vi "Check for Rx Label Updates.vi"(8 "error in":errorcluster, 9 "labels settings for RT":T1[](array[typedef]) {"Label Timestamp Channel Data Reference" format="%.0x"; "Word Initial Raw Value" format="%032.0f"; "Label Disable/Trigger Channel Reference" format="%.0x"; "parameter driver data"."Tx parameter refs" format="%.0x"; "SDI" format="%02b"; "label" format="%.0o"}, 10 "channel number in":u8, 11 "board handle in":u8) -> (0 "error out":errorcluster, 1 "labels updated?":bool[](array[boolean]), 2 "channel number out":u8, 3 "board handle out":u8)   [LabVIEW 2024, in "AIM ARINC 429 Hardware API.lvlib"]
uses:
  AIM ARINC 429 Hardware API.lvlib
  Shared/RT Label Settings.ctl
  Shared/Label.ctl
  Shared/RT Parameters.ctl
  Shared/Parameter Definition.ctl
  <vilib>/NI/NI VeriStand Encoding and Decoding/Encoding.ctl
  <vilib>/NI VeriStand/Custom Device API/Custom Device Item Ref.ctl
  Shared/Transfer Type.ctl
  <vilib>/NI VeriStand/Custom Device API/Data Reference.ctl
  <instrlib>/AIM GmbH/_ARINC-429/subvi/Error Converter (ErrCode or Status).vi
  <instrlib>/AIM GmbH/_ARINC-429/subvi/Get Library Path.vi
  <instrlib>/AIM GmbH/_ARINC-429/VIs/Library/Api429Lib Error Desc Get.vi
  <instrlib>/AIM GmbH/_ARINC-429/subvi/Get Error Number Offset.vi
  <vilib>/Utility/error.llb/Error Cluster From Error Code.vi
  <instrlib>/AIM GmbH/_ARINC-429/AIM429LV.lvlib
  <vilib>/NI/NI VeriStand Encoding and Decoding/Encoding and Decoding.lvlib
  <vilib>/NI VeriStand/Custom Device API/Custom Device API.lvlib
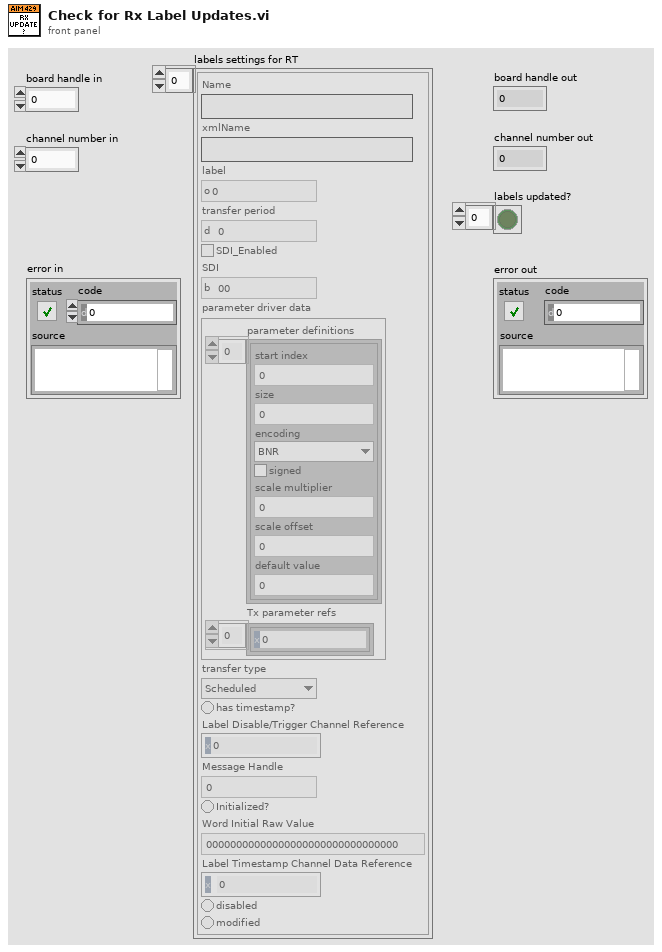
[diagram p1: front panel]
types:
  T1 = typedef "RT Label Settings.ctl" = cluster{"Name":string, "xmlName":string, "label":T2, "transfer period":u32, "SDI_Enabled":bool, "SDI":u8, "parameter driver data":T3, "transfer type":T7, "has timestamp?":bool, "Label Disable/Trigger Channel Reference":T6, "Message Handle":u64, "Initialized?":bool, "Word Initial Raw Value":u32, "Label Timestamp Channel Data Reference":T8, "disabled":bool, "modified":bool}
  T2 = typedef "Label.ctl" = u8
  T3 = typedef "RT Parameters.ctl" = cluster{"parameter definitions":T4[], "Tx parameter refs":T6[]}
  T4 = typedef "Parameter Definition.ctl" = cluster{"start index":i32, "size":i32, "encoding":T5, "signed":bool, "scale multiplier":dbl, "scale offset":dbl, "default value":dbl}
  T5 = typedef "Encoding and Decoding.lvlib/Encoding.ctl" = enum16{"BNR", "BCD", "Discrete"}
  T6 = typedef "Custom Device API.lvlib/Custom Device Item Ref.ctl" = u64
  T7 = typedef "Transfer Type.ctl" = enum16{"Scheduled", "Acyclic", "Block", "Strobe"}
  T8 = typedef "Custom Device API.lvlib/Data Reference.ctl" = i32
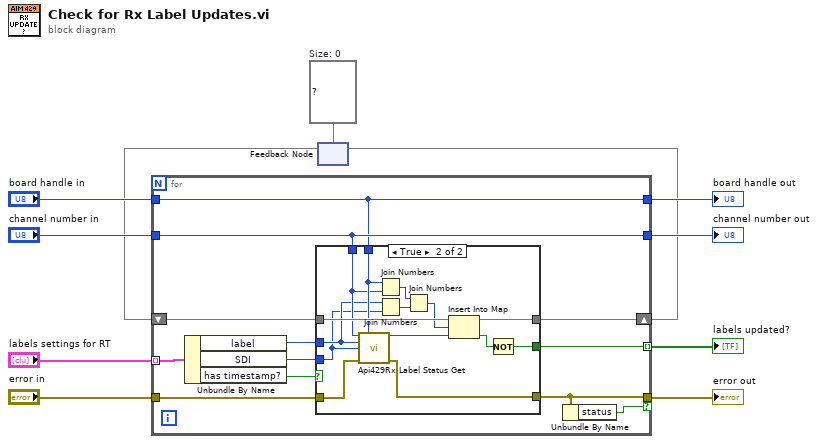
[diagram p0: block diagram]
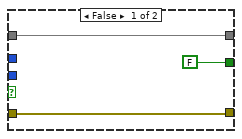
[diagram p2: hidden frame]
diagram:
  w4 = map{u32, i32} {}  # Size: 0
  n1 = feedback #1(w4) -> (w3:map{u32, i32})
  n2 = for {
    tunnel: "board handle in" -> [w18]
    tunnel: "channel number in" -> [w19]
    tunnel: "labels settings for RT" -> [w23] mode=indexing
    tunnel: [w19] -> w6
    tunnel: [w18] -> w5
    shift-right: [w15] -> w2
    shift-left: w3 -> [w16]
    tunnel: [w14] -> w1 mode=indexing
    tunnel: "error in" -> [w20]
    tunnel: [w13] -> w7 if=w12
    n3 = Unbundle By Name(w23) -> ("label"=w22:T2, "SDI"=w21:u8, "has timestamp?"=w17:bool)
    n4 = case shown="True" w17 {
      tunnel: w22 -> [_ w31]
      tunnel: w21 -> [_ w30]
      tunnel: w20 -> [w26 w40]
      tunnel: [w26 w39] -> w13
      tunnel: w19 -> [_ w32]
      tunnel: w18 -> [_ w33]
      tunnel: w16 -> [w24 w37]
      tunnel: [w24 w36] -> w15
      tunnel: [FALSE w34] -> w14
      frame False {
      }
      frame True {
        n5 = call <instrlib>:"Api429Rx Label Status Get.vi"("b_Chn"=w32, "board_handle"=w33, "b_Label"=w31, "b_Sdi"=w30, "error in (no error)"=w40) -> ("px_LabCnt out"=w38:u32, "error out"=w39:errorcluster)  [unwired: 7 in, 2 out]
        n6 = Join Numbers(hi=w33, lo=w32) -> ((hi.lo)=w28:u16)
        n7 = Join Numbers(hi=w31, lo=w30) -> ((hi.lo)=w29:u16)
        n8 = Join Numbers(hi=w28, lo=w29) -> ((hi.lo)=w27:u32)
        n9 = Insert Into Map(map in=w37, key=w27, value=w38) -> (map out=w36:map{u32, i32}, value unchanged?=w35:bool)  [unwired: 1 out]
        n10 = Not(x=w35) -> (.not. x?=w34:bool)
      }
    }
    n11 = Unbundle By Name(w13) -> ("status"=w12:bool)
  }
  "board handle out" <- w5
  "channel number out" <- w6
  "error out" <- w7
  "labels updated?" <- w1
  n12 = feedback-in #1(w2) -> ()
